vi "Network-Order Bytes To Words U16.vi"(1 "bytes in":u8[](array[numeric]) format="%02x") -> (0 "words out":u16[](array[numeric]) format="%x")   [LabVIEW 2020, in "NI_Bit Manipulation.lvlib"]
uses:
  <vilib>/Bit Manipulation/NI_Bit Manipulation.lvlib
  445b2e95-4c26-4098-854f-89dad29dbcf2.vi
  445b2e95-4c26-4098-854f-89dad29dbcf2.vi/6b904183-ac25-4398-9280-d06e18482e71.vi
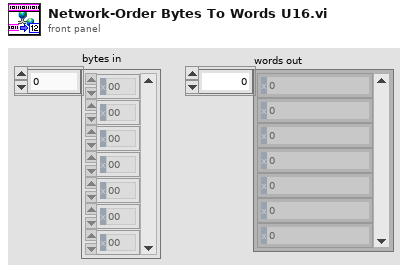
[diagram p1: front panel]
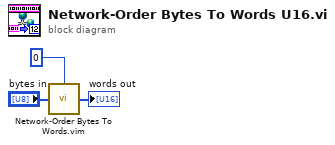
[diagram p0: block diagram]
diagram:
  n1 = call "Network-Order Bytes To Words.vim"("bytes in"="bytes in", "word type"=u16 0) -> ("words out"=→"words out":u16[])
